vi "Joystick Monitor.vi"() -> ()   [LabVIEW 2012]
uses:
  <vilib>/Utility/inputDevices.llb/closeJoystick.vi
  <vilib>/Utility/inputDevices.llb/joystickAcquire.vi
panel:
  in  "loop rate (ms)":u32(knob)=10 min=5 max=100 step=5 scale=0.0..100.0
  out "XY Graph":cluster{i32[], i32[]}(graph)
  in  "axis info":T1
  out "button info":T2
  in  "stop":bool
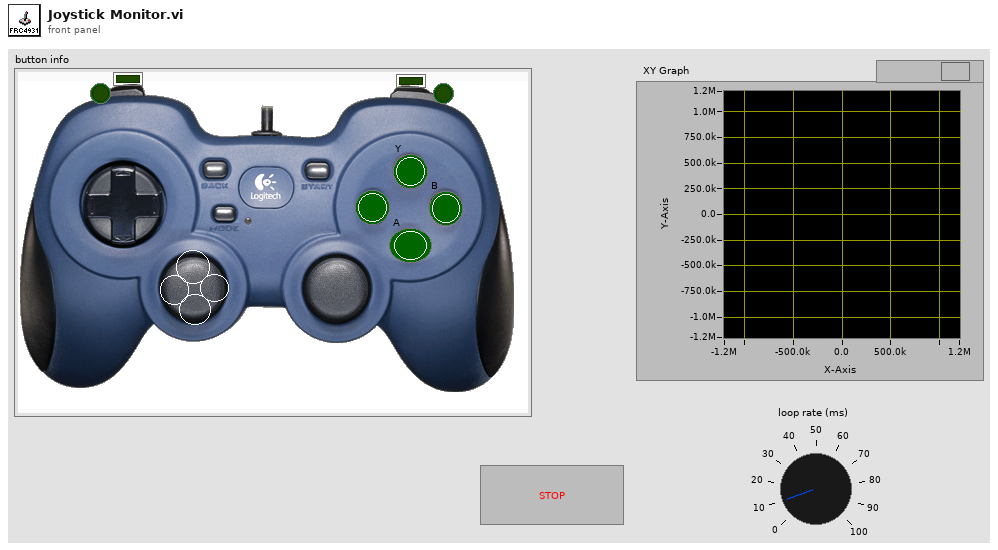
[diagram p1: front panel]
types:
  T1 = cluster{"X axis":i32, "Y axis":i32, "Z axis":i32, "X axis rotation":i32, "Y axis rotation":i32, "Z axis rotation":i32, "U axis":i32, "V axis":i32}
  T2 = cluster{"X":bool, "A":bool, "B":bool, "Y":bool, "LB":bool, "RB":bool, "LT":bool, "RT`":bool, "button 9":bool, "button 10":bool, "-X":bool, "+X":bool, "+Y":bool, "-Y":bool, "button 15":bool, "button 16":bool, "button 17":bool, "button 18":bool, "button 19":bool, "button 20":bool, "button 21":bool, "button 22":bool, "button 23":bool, "button 24":bool, "button 25":bool, "button 26":bool, "button 27":bool, "button 28":bool, "button 29":bool, "button 30":bool, "button 31":bool, "button 32":bool}
  T3 = cluster{"X":bool, "A":bool, "B":bool, "Y":bool, "LB":bool, "RB":bool, "LT":bool, "RT`":bool, "button 9":bool, "button 10":bool, "button 11":bool, "button 12":bool, "button 13":bool, "button 14":bool, "button 15":bool, "button 16":bool, "button 17":bool, "button 18":bool, "button 19":bool, "button 20":bool, "button 21":bool, "button 22":bool, "button 23":bool, "button 24":bool, "button 25":bool, "button 26":bool, "button 27":bool, "button 28":bool, "button 29":bool, "button 30":bool, "button 31":bool, "button 32":bool}
  T4 = cluster{"button 1":bool, "button 2":bool, "button 3":bool, "button 4":bool, "button 5":bool, "button 6":bool, "button 7":bool, "button 8":bool, "button 9":bool, "button 10":bool, "button 11":bool, "button 12":bool, "button 13":bool, "button 14":bool, "button 15":bool, "button 16":bool, "button 17":bool, "button 18":bool, "button 19":bool, "button 20":bool, "button 21":bool, "button 22":bool, "button 23":bool, "button 24":bool, "button 25":bool, "button 26":bool, "button 27":bool, "button 28":bool, "button 29":bool, "button 30":bool, "button 31":bool, "button 32":bool}
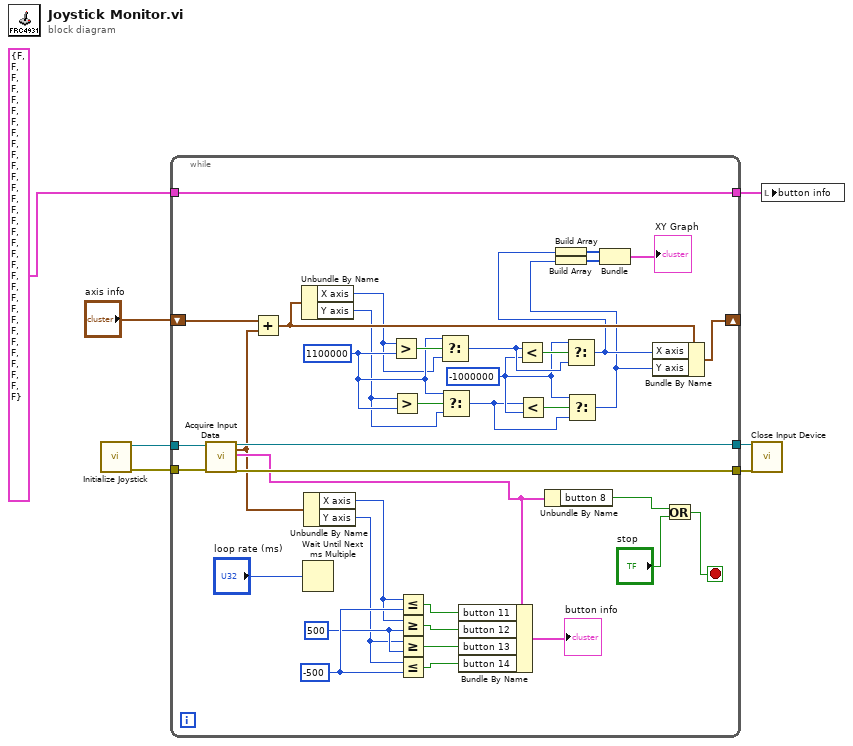
[diagram p0: block diagram]
diagram:
  n1 = call <vilib>:"Initialize Joystick.vi"() -> ("error out"=w6:errorcluster, "device ID"=w7:refnum<k1>)  [unwired: 10 in]
  n2 = while {
    tunnel: w7 -> [w45]
    tunnel: w6 -> [w44]
    tunnel: [w43] -> w5
    tunnel: [w42] -> w4
    shift-right: [w31] -> _
    shift-left: "axis info" -> [w40]
    tunnel: T3 {"X"=FALSE, "A"=FALSE, "B"=FALSE, "Y"=FALSE, "LB"=FALSE, "RB"=FALSE, "LT"=FALSE, "RT`"=FALSE, "button 9"=FALSE, "button 10"=FALSE, "button 11"=FALSE, "button 12"=FALSE, "button 13"=FALSE, "button 14"=FALSE, "button 15"=FALSE, "button 16"=FALSE, "button 17"=FALSE, "button 18"=FALSE, "button 19"=FALSE, "button 20"=FALSE, "button 21"=FALSE, "button 22"=FALSE, "button 23"=FALSE, "button 24"=FALSE, "button 25"=FALSE, "button 26"=FALSE, "button 27"=FALSE, "button 28"=FALSE, "button 29"=FALSE, "button 30"=FALSE, "button 31"=FALSE, "button 32"=FALSE} ("button info") -> [w21]
    tunnel: [w21] -> w1
    stop <- w23 stop-if-true
    w19 = 500 ("y")
    w20 = -500 ("y")
    w34 = -1000000 ("y")
    w33 = 1100000 ("y")
    n3 = call-poly <vilib>:"Acquire Input Data.vi"("device ID"=w45, "error in (no error)"=w44) -> ("device ID"=w43:refnum<k1>, "axis info"=w10:T1, "button info"=w12:T4, "error out"=w42:errorcluster)  [unwired: 13 in, 1 out]
    n4 = Add(x=w40, y=w10) -> (x+y=w30:T1)
    n5 = Unbundle By Name(w30) -> ("X axis"=w14:i32, "Y axis"=w17:i32)
    n6 = Wait Until Next ms Multiple(millisecond multiple="loop rate (ms)") -> ()  [unwired: 1 out]
    n7 = Unbundle By Name(w10) -> ("X axis"=w9:i32, "Y axis"=w8:i32)
    n8 = Greater?(x=w14, y=w33) -> (0:w39:bool)
    n9 = Greater?(x=w17, y=w33) -> (0:w38:bool)
    n10 = Less Or Equal?(x=w9, y=w20) -> (x <= y?=w15:bool)
    n11 = Greater Or Equal?(x=w9, y=w19) -> (x >= y?=w13:bool)
    n12 = Greater Or Equal?(x=w8, y=w19) -> (x >= y?=w18:bool)
    n13 = Less Or Equal?(x=w8, y=w20) -> (x <= y?=w16:bool)
    n14 = Select(t=w33, s=w39, f=w14) -> (s? t:f=w35:i32)
    n15 = Select(t=w33, s=w38, f=w17) -> (s? t:f=w32:i32)
    n16 = Bundle By Name(cluster=w12, "button 11"=w15, "button 12"=w13, "button 13"=w18, "button 14"=w16) -> (→"button info":T4)
    n17 = Less?(x=w35, y=w34) -> (x < y?=w37:bool)
    n18 = Less?(x=w32, y=w34) -> (x < y?=w36:bool)
    n19 = Unbundle By Name(w12) -> ("button 8"=w22:bool)
    n20 = Select(t=w34, s=w37, f=w35) -> (s? t:f=w29:i32)
    n21 = Build Array(w29) -> (w28:i32[])
    n22 = Select(t=w34, s=w36, f=w32) -> (s? t:f=w27:i32)
    n23 = Build Array(w27) -> (w26:i32[])
    n24 = Bundle(w28, w26) -> (→"XY Graph":cluster{i32[], i32[]})  [unwired: 1 in]
    n25 = Bundle By Name(cluster=w30, "X axis"=w29, "Y axis"=w27) -> (w31:T1)
    n26 = Or(x=w22, y="stop") -> (x .or. y?=w23:bool)
  }
  n27 = call-poly <vilib>:"Close Input Device.vi"("error in (no error)"=w4, "device ID"=w5) -> ()  [unwired: 8 in, 1 out]
  n28 = local write "button info"(w1) -> ()
